vi "Wheel Separation to Frame Positions.vi"(10 "wheel separation length":dbl=1.5, 11 "wheel separation width":dbl=1.0) -> (0 "wheel y positions":dbl[](array[numeric]), 1 "wheel x positions":dbl[](array[numeric]), 2 "coerced wheel separation length":dbl, 3 "coerced wheel separation width":dbl, 4 "wheel frame angles (rad)":dbl[](array[numeric]), 6 "wheel indexes":i32[](array[numeric]))   [LabVIEW 2017, in "NI_Robotics_Ackermann Steering Frame.lvclass"]
uses:
  <vilib>/robotics/Steering/Ackermann Steering Frame/NI_Robotics_Ackermann Steering Frame.lvclass
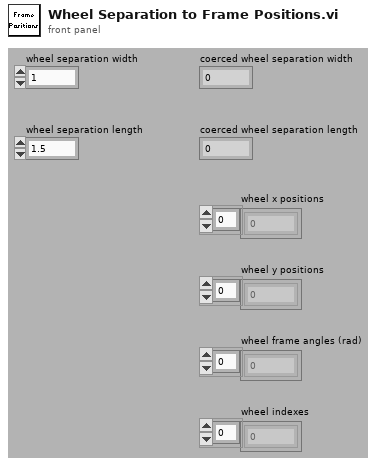
[diagram p1: front panel]
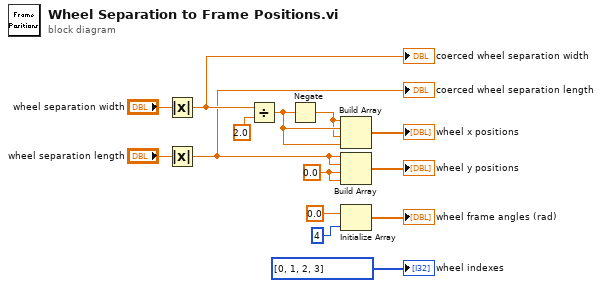
[diagram p0: block diagram]
diagram:
  w9 = 0.0 ("element")
  n1 = Absolute Value(x="wheel separation width") -> (abs(x)=w14:dbl)
  "coerced wheel separation width" <- w14
  n2 = Absolute Value(x="wheel separation length") -> (abs(x)=w1:dbl)
  "coerced wheel separation length" <- w1
  n3 = Divide(x=w14, y=2.0) -> (x/y=w12:dbl)
  n4 = Negate(x=w12) -> (-x=w8:dbl)
  n5 = Build Array(w8, w12, w8, w12) -> (→"wheel x positions":dbl[])
  n6 = Build Array(w1, w1, w9, w9) -> (→"wheel y positions":dbl[])
  n7 = Initialize Array(0.0 ("element"), 4 ("dimension size")) -> (→"wheel frame angles (rad)":dbl[])
  "wheel indexes" <- i32[] [0, 1, 2, 3] ("wheel indexes")
